vi "1b - Local variable.vi"() -> ()   [LabVIEW 2010]
panel:
  in  "stop":bool
  out "Chart 3":i32(graph)
  out "Chart 2":dbl(graph)
  out "Chart 1":dbl(graph)
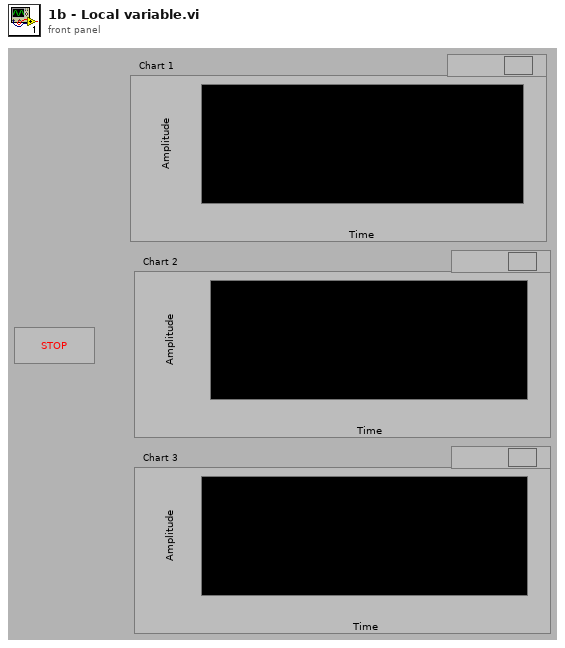
[diagram p1: front panel]
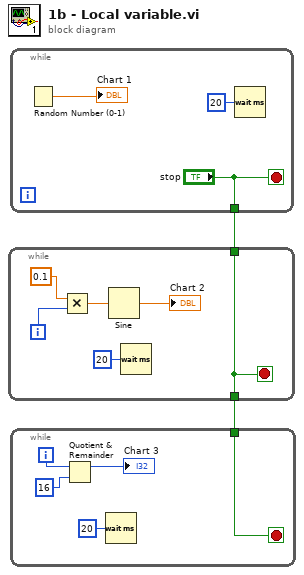
[diagram p0: block diagram]
diagram:
  n1 = while {
    tunnel: ["stop"] -> w2
    stop <- "stop" stop-if-true
    n2 = Random Number (0-1)() -> (number: 0 to 1=→"Chart 1":dbl)
    n3 = Wait (ms)(milliseconds to wait=u32 20) -> ()  [unwired: 1 out]
  }
  n4 = while {
    tunnel: w2 -> [w6]
    tunnel: [w6] -> w1
    i -> [w9]
    stop <- w6 stop-if-true
    n5 = Multiply(x=0.1, y=w9) -> (x*y=w8:dbl)
    n6 = Sine(x=w8) -> (sin(x)=→"Chart 2":dbl)
    n7 = Wait (ms)(milliseconds to wait=u32 20) -> ()  [unwired: 1 out]
  }
  n8 = while {
    tunnel: w1 -> [w12]
    i -> [w15]
    stop <- w12 stop-if-true
    n9 = Quotient & Remainder(x=w15, y=16) -> (x-y*floor(x/y)=→"Chart 3":i32)  [unwired: 1 out]
    n10 = Wait (ms)(milliseconds to wait=u32 20) -> ()  [unwired: 1 out]
  }
